vi "SHRHA Specific Heat Ratio of Humid Air.vi"(1 "Gas Presure":dbl[unit]=80000.0 min=80000.0 max=120000.0, 2 "Tceg":dbl[unit], 3 "RH":dbl) -> (0 "SHRHA":dbl)   [LabVIEW 2018]
panel:
  out "SHRHA\nSpecific Heat ratio of Humid Air\nSHRHA=SHCHA/(SHCHA-R)":dbl(knob) scale=0.0..1.5
  out "Temprature Of Input Air\nKelvin Degree":dbl[unit](slide) scale=273.0..373.0
  out "Tk":dbl[unit]
  out "Temprature Of Input Air\nCentigrade Degree":dbl[unit](slide) scale=0.0..100.0
  out "Humidity of Input Air":dbl(knob) scale=0.0..100.0
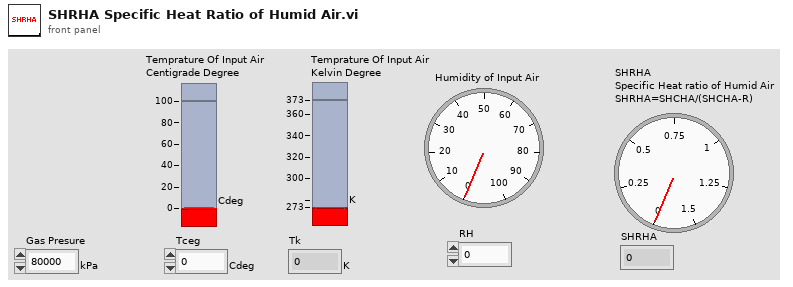
[diagram p1: front panel]
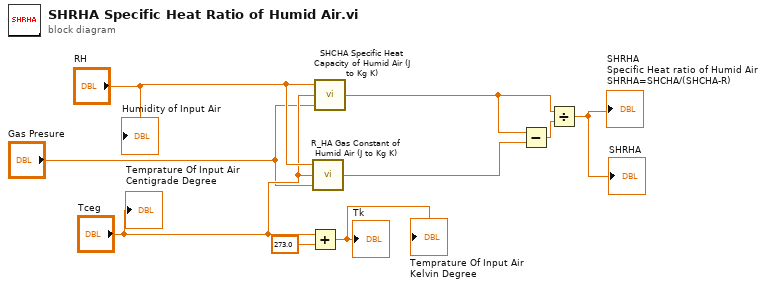
[diagram p0: block diagram]
diagram:
  n1 = Add(x="Tceg", y=dbl[unit] 273.0) -> (x+y=→"Tk" →"Temprature Of Input Air\nKelvin Degree":dbl[unit])
  n2 = call "R_HA Gas Constant of Humid Air (J to Kg K).vi"("Gas Presure"="Gas Presure", "Tceg"="Tceg", "RH"="RH") -> ("R_HA"=w5:dbl[unit])
  n3 = call "SHCHA Specific Heat Capacity of Humid Air (J to Kg K).vi"("Gas Presure"="Gas Presure", "Tceg"="Tceg", "RH"="RH") -> ("SHCHA"=w4:dbl[unit])
  n4 = Subtract(x=w4, y=w5) -> (x-y=w6:dbl[unit])
  n5 = Divide(x=w4, y=w6) -> (x/y=→"SHRHA\nSpecific Heat ratio of Humid Air\nSHRHA=SHCHA/(SHCHA-R)" →"SHRHA":dbl)
  "Humidity of Input Air" <- "RH"
  "Temprature Of Input Air\nCentigrade Degree" <- "Tceg"
